vi "11-2.vi"() -> ()   [LabVIEW 2019, in "11.lvlib"]
uses:
  11.lvlib
panel:
  out "Sync Step":i32
  out "Flashes":u64
  out "Octo":i16[][](array[ring])
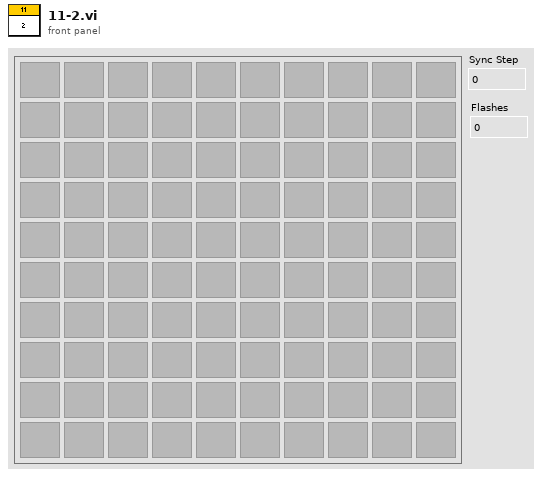
[diagram p1: front panel]
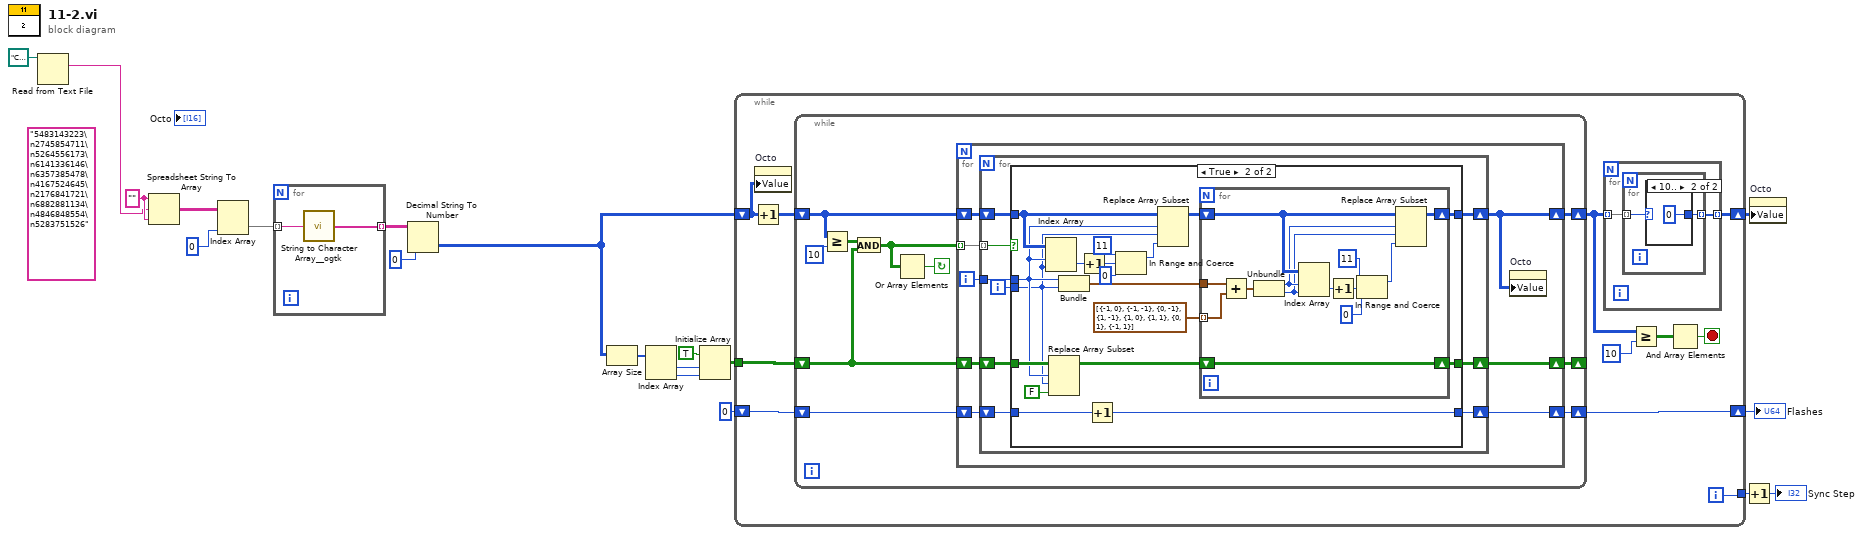
[diagram p0: block diagram]
diagram:
  w19 = "" ("format string")
  (unwired) "5483143223\n2745854711\n5264556173\n6141336146\n6357385478\n4167524645\n2176841721\n6882881134\n4846848554\n5283751526"
  n1 = Read from Text File(file (use dialog)=path "C:/Users/craig.walker/Documents/GitHub/lv2019-Advent-of-Code-2021/11/input.txt") -> (text=w2:string)  [unwired: 3 in, 3 out]
  n2 = Spreadsheet String To Array(format string=w19, spreadsheet string=w2, array type (2D Dbl)=w19) -> (array=w18:string[][])  [unwired: 1 in]
  n3 = Index Array(array=w18, index (col)=0 ("disabled index (col)")) -> (element=w16:string[])  [unwired: 1 in]
  n4 = for {
    tunnel: w16 -> [w21] mode=indexing
    tunnel: [w20] -> w15 mode=indexing
    n5 = call <userlib>:"String to Character Array__ogtk.vi"("Input String"=w21) -> ("Character Array"=w20:string[])
  }
  n6 = Decimal String To Number(string=w15, default (0L)=i16 0 ("Octo")) -> (number=w13:i16[][])  [unwired: 1 in, 1 out]
  n7 = Array Size(array=w13) -> (size(s)=w12:i32[])
  n8 = Index Array(array=w12) -> (element #1=w11:i32, element #2=w10:i32)  [unwired: 2 in]
  n9 = Initialize Array(TRUE, w11, w10) -> (w8:bool[][])
  n10 = while {
    shift-right: [w25] -> w1
    shift-left: w13 -> [w24]
    tunnel: w8 -> [w22]
    shift-right: [w31] -> w6
    shift-left: u64 0 -> [w32]
    tunnel: [w26] -> w4
    i -> [w26]
    stop <- w27 stop-if-true
    n11 = Increment(x=w24) -> (x+1=w23:i16[][])
    n12 = property on="Octo" class="Arr (strict)"("Value"=w24) -> ()  [unwired: 2 in, 2 out]
    n13 = while {
      shift-right: [w39] -> w30
      shift-left: w23 -> [w42]
      shift-right: [w35] -> _
      shift-left: w22 -> [w36]
      shift-right: [w33] -> w31
      shift-left: w32 -> [w34]
      stop <- w40 continue-if-true
      n14 = Greater Or Equal?(x=w42, y=i16 10) -> (x >= y?=w38:bool[][])
      n15 = And(x=w38, y=w36) -> (x .and. y?=w37:bool[][])
      n16 = Or Array Elements(Boolean array=w37) -> (logical OR=w40:bool)
      n17 = for {
        tunnel: w37 -> [w50] mode=indexing
        shift-right: [w47] -> w39
        shift-left: w42 -> [w49]
        shift-right: [w43] -> w35
        shift-left: w36 -> [w46]
        shift-right: [w44] -> w33
        shift-left: w34 -> [w45]
        i -> [w48]
        n18 = for {
          tunnel: w50 -> [w59] mode=indexing
          tunnel: w48 -> [w57]
          shift-right: [w55] -> w47
          shift-left: w49 -> [w58]
          shift-right: [w53] -> w43
          shift-left: w46 -> [w54]
          shift-right: [w51] -> w44
          shift-left: w45 -> [w52]
          i -> [w56]
          n19 = case shown="True" w59 {
            tunnel: w58 -> [w62 w78]
            tunnel: w57 -> [_ w74]
            tunnel: w56 -> [_ w73]
            tunnel: [w62 w66] -> w55
            tunnel: w54 -> [w61 w76]
            tunnel: [w61 w67] -> w53
            tunnel: w52 -> [w60 w65]
            tunnel: [w60 w64] -> w51
            frame False {
            }
            frame True {
              n20 = Index Array(array=w78, index (row)=w74, index (col)=w73) -> (element=w79:i16)
              n21 = Replace Array Subset(array=w76, new element=FALSE ("new element/subarray"), index (row)=w74, index (col)=w73) -> (w75:bool[][])
              n22 = Bundle(w74, w73) -> (w80:cluster{i32, i32})  [unwired: 1 in]
              n23 = Increment(x=w79) -> (x+1=w69:i16)
              n24 = Increment(x=w65) -> (x+1=w64:u64)
              n25 = In Range and Coerce(upper limit=i16 11, x=w69, lower limit=i16 0) -> (coerced(x)=w68:i16)  [unwired: 1 out]
              n26 = Replace Array Subset(array=w78, new element=w68, index (row)=w74, index (col)=w73) -> (w77:i16[][])
              n27 = for {
                tunnel: cluster{"Row":i32, "Col":i32}[] [{"Row"=-1, "Col"=0}, {"Row"=-1, "Col"=-1}, {"Row"=0, "Col"=-1}, {"Row"=1, "Col"=-1}, {"Row"=1, "Col"=0}, {"Row"=1, "Col"=1}, {"Row"=0, "Col"=1}, {"Row"=-1, "Col"=1}] -> [w92] mode=indexing
                tunnel: w80 -> [w93]
                shift-right: [w84] -> w66
                shift-left: w77 -> [w85]
                shift-right: [w81] -> w67
                shift-left: w75 -> [w81]
                n28 = Add(x=w93, y=w92) -> (x+y=w91:cluster{i32, i32})
                n29 = Unbundle(w91) -> (w83:i32, w82:i32)
                n30 = Index Array(array=w85, index (row)=w83, index (col)=w82) -> (element=w90:i16)
                n31 = Increment(x=w90) -> (x+1=w87:i16)
                n32 = In Range and Coerce(upper limit=i16 11, x=w87, lower limit=i16 0) -> (coerced(x)=w86:i16)  [unwired: 1 out]
                n33 = Replace Array Subset(array=w85, new element=w86, index (row)=w83, index (col)=w82) -> (w84:i16[][])
              }
            }
          }
        }
        n34 = property on="Octo" class="Arr (strict)"("Value"=w47) -> ()  [unwired: 2 in, 2 out]
      }
    }
    n35 = for {
      tunnel: w30 -> [w95] mode=indexing
      tunnel: [w94] -> w25 mode=indexing
      n36 = for {
        tunnel: w95 -> [w97] mode=indexing
        tunnel: [w96] -> w94 mode=indexing
        n37 = case shown="10.." w97 {
          selector: w97 -> [w98 _]
          tunnel: [w98 i16 0 ("String")] -> w96
          frame 0, Default {
          }
          frame 10.. {
          }
        }
      }
    }
    n38 = Greater Or Equal?(x=w30, y=i16 10 ("upper limit")) -> (x >= y?=w28:bool[][])
    n39 = And Array Elements(Boolean array=w28) -> (logical AND=w27:bool)
  }
  "Flashes" <- w6
  n40 = Increment(x=w4) -> (x+1=→"Sync Step":i32)
  n41 = property on="Octo" class="Arr (strict)"("Value"=w1) -> ()  [unwired: 2 in, 2 out]
